vi "ConvertCoordinates (1).vi"(2 "Target Coordinate (mm)":dbl min=0.0, 3 "Start Coordinate (mm)":dbl) -> (0 "Direction":dbl, 1 "Distance To Move (mm)":dbl)   [LabVIEW 2013]
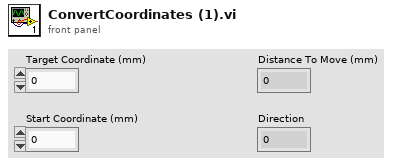
[diagram p1: front panel]
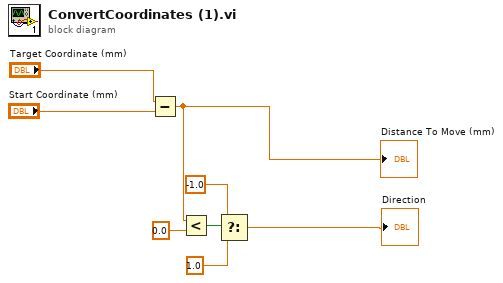
[diagram p0: block diagram]
diagram:
  n1 = Subtract(x="Target Coordinate (mm)", y="Start Coordinate (mm)") -> (x-y=w3:dbl)
  "Distance To Move (mm)" <- w3
  n2 = Less?(x=w3, y=0.0) -> (x < y?=w5:bool)
  n3 = Select(t=-1.0, s=w5, f=1.0) -> (s? t:f=→"Direction":dbl)
